vi "DamnYankeeFPGA.vi"() -> ()   [LabVIEW 2013]
doc: "This is the Damn Yankee FPGA code, at the moment it is only being used to read in the values from the remote control. We're using the FPGA to read a PWM signal because doing it in RT wasn't consistent enough.\n\nEric Schneider, May 2014"
uses:
  <vilib>/rvi/Emulation/niFpgaSctlEmulationGetInTimedLoop.vi
  <vilib>/rvi/Emulation/niFpgaEmulationReportErrorSimple.vi
  <vilib>/rvi/Emulation/niFpgaGetClockAttributes.vi
  <vilib>/rvi/eio/common/nirviEmuTemplateMethod_errors.vi
  <vilib>/rvi/Emulation/niFpgaCriticalErrorInLSC.vi
  <vilib>/eio/EIONode/EIONode.xnode
panel:
  out "ConnectorA/DIO2":bool
  out "ConnectorA/DIO1":bool
  out "Sail ratio":sgl
  out "Rudder ratio":sgl
  out "Switch ratio":sgl
  out "Counter Out":i16
  out "High Counter Out":i16
  out "ConnectorA/DIO0":bool
  out "Counter In":i16
  out "High Counter In":i16
  out "Loop counter":i32
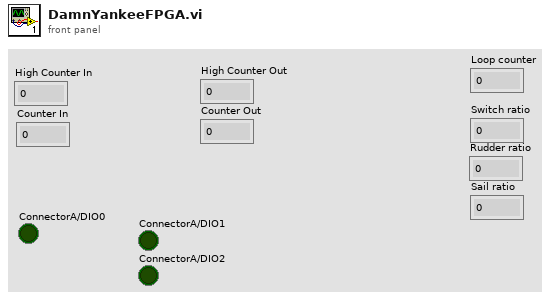
[diagram p1: front panel]
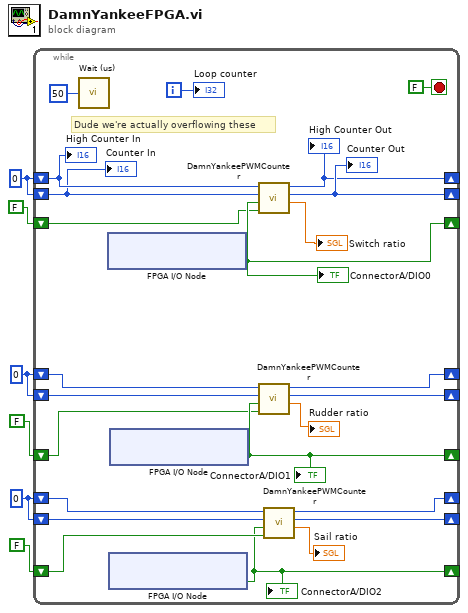
[diagram p0: block diagram]
diagram:
  w2 = i16 0 ("High Counter Out")
  w4 = i16 0 ("High Counter Out")
  w6 = i16 0 ("High Counter Out")
  n1 = while {
    shift-right: [w10] -> _
    shift-left: w6 -> [w30]
    shift-right: [w26] -> _
    shift-left: w6 -> [w29]
    shift-right: [w28] -> _
    shift-left: FALSE ("Jumped Up Out") -> [w27]
    shift-right: [w22] -> _
    shift-left: w4 -> [w21]
    shift-right: [w20] -> _
    shift-left: w4 -> [w19]
    shift-right: [w18] -> _
    shift-left: FALSE ("Jumped Up Out") -> [w17]
    shift-right: [w12] -> _
    shift-left: w2 -> [w13]
    shift-right: [w14] -> _
    shift-left: w2 -> [w15]
    shift-right: [w11] -> _
    shift-left: FALSE ("Jumped Up Out") -> [w16]
    i -> [w24]
    stop <- FALSE stop-if-true
    # "Dude we're actually overflowing these"
    n2 = call "Wait (us)"("Count(uSec)"=u32 50) -> ()  [unwired: 1 out]
    n3 = xnode "FPGA I/O Node"() -> ("ConnectorA/DIO0"=w28:bool)  [unwired: 1 in, 1 out]
    "ConnectorA/DIO0" <- w28
    n4 = xnode "FPGA I/O Node"() -> ("ConnectorA/DIO2"=w11:bool)  [unwired: 1 in, 1 out]
    "ConnectorA/DIO2" <- w11
    n5 = xnode "FPGA I/O Node"() -> ("ConnectorA/DIO1"=w18:bool)  [unwired: 1 in, 1 out]
    "ConnectorA/DIO1" <- w18
    n6 = call "DamnYankeePWMCounter.vi"("Old Value"=w27, "New Value"=w28, "Total Ticks In"=w29, "Ticks High In"=w30) -> ("Ratio"=→"Switch ratio":sgl, "Ticks Total Out"=w26:i16, "Ticks High Out"=w10:i16)  [unwired: 5 in]
    "High Counter Out" <- w10
    "Counter Out" <- w26
    n7 = call "DamnYankeePWMCounter.vi"("Old Value"=w17, "New Value"=w18, "Total Ticks In"=w19, "Ticks High In"=w21) -> ("Ratio"=→"Rudder ratio":sgl, "Ticks Total Out"=w20:i16, "Ticks High Out"=w22:i16)  [unwired: 5 in]
    n8 = call "DamnYankeePWMCounter.vi"("Old Value"=w16, "New Value"=w11, "Total Ticks In"=w15, "Ticks High In"=w13) -> ("Ratio"=→"Sail ratio":sgl, "Ticks Total Out"=w14:i16, "Ticks High Out"=w12:i16)  [unwired: 5 in]
    "Loop counter" <- w24
    "High Counter In" <- w30
    "Counter In" <- w29
  }
